vi "Child Inheritance.vi"(8 "error in (no error)":errorcluster, 10 "Child In":refnum<class "Circular Buffer.lvclass">, 11 "Parent In":refnum<class "Circular Buffer.lvclass">) -> (0 "error out":errorcluster, 2 "Child Out":refnum<class "Circular Buffer.lvclass">, 3 "Parent Out":refnum<class "Circular Buffer.lvclass">)   [LabVIEW 2024, in "Circular Buffer.lvclass"]
uses:
  Circular Buffer.lvclass
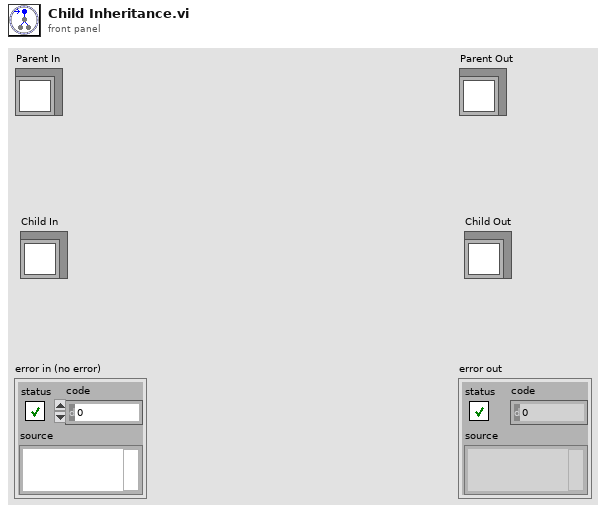
[diagram p1: front panel]
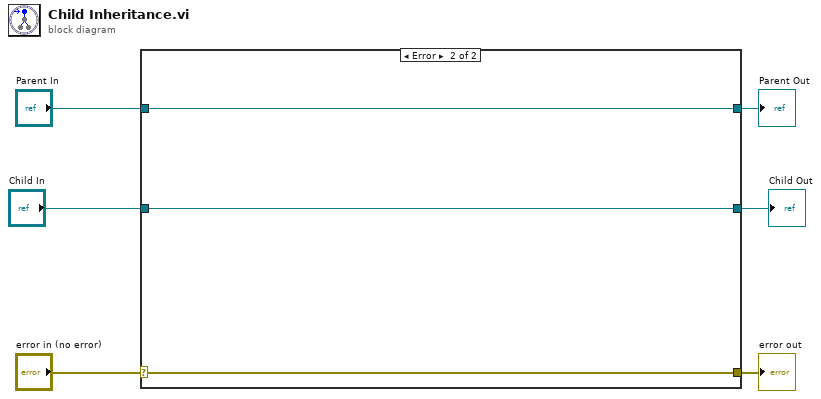
[diagram p0: block diagram]
diagram:
  n1 = case shown="Error" "error in (no error)" {
    selector: "error in (no error)" -> [w8 w12]
    tunnel: [w8 w12] -> w5
    tunnel: [w9 w11] -> w3
    tunnel: "Parent In" -> [w9 w11]
    tunnel: [w7 w10] -> w2
    tunnel: "Child In" -> [w7 w10]
    frame No Error {
      # "Wire the error cluster across even in the \"No Error\"\ncase so that warnings get propagated."
    }
    frame Error {
    }
  }
  "error out" <- w5
  "Parent Out" <- w3
  "Child Out" <- w2
